vi "general.ascii2hex.vi"(11 "Ascii input Message":string="0") -> (3 "Hex output Message":string="0")   [LabVIEW 2011]
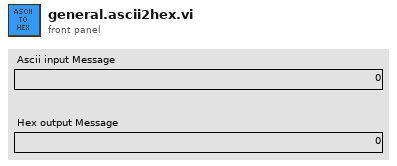
[diagram p1: front panel]
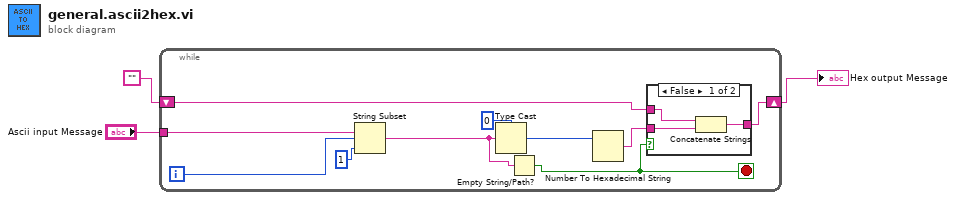
[diagram p0: block diagram]
diagram:
  n1 = while {
    shift-right: [w6] -> w2
    shift-left: "" -> [w8]
    tunnel: "Ascii input Message" -> [w4]
    i -> [w11]
    stop <- w5 stop-if-true
    n2 = String Subset(string=w4, offset (0)=w11, length (rest)=1 ("length (rest)")) -> (substring=w9:string)
    n3 = Type Cast(type=u8 0, x=w9) -> (*(type *) &x=w12:u8)
    n4 = Empty String/Path?(string/path=w9) -> (empty?=w5:bool)
    n5 = Number To Hexadecimal String(2:w12) -> (0:w7:string)  [unwired: 1 in]
    n6 = case shown="False" w5 {
      tunnel: w8 -> [w16 w17]
      tunnel: w7 -> [w15 _]
      tunnel: [w14 w17] -> w6
      frame False {
        n7 = Concatenate Strings(w16, w15) -> (w14:string)
      }
      frame True {
      }
    }
  }
  "Hex output Message" <- w2
